vi "Custom Aggregation (1D DBL Array).vi"(0 "data in":dbl[](array[numeric]), 1 "reset? (F)":bool, 5 "aggregation settings":T1={"interval"=1, "interval unit"=enum."Runs", "synchronization of intervals"=enum."Not synchronized", "algorithm"=enum."Average"}, 9 "system info in":refnum<class "EP System Info.lvclass">, 11 "error in (no error)":errorcluster, 12 "data timestamp":timestamp) -> (4 "aggregated minimum values":dbl[](array[numeric]), 6 "aggregated averaged/RMS values":dbl[](array[numeric]), 8 "aggregated maximum values":dbl[](array[numeric]), 10 "system info out":refnum<class "EP System Info.lvclass">, 13 "aggregated data valid?":bool, 14 "aggregated data timestamp":timestamp, 15 "error out":errorcluster)   [LabVIEW 2014, in "NI_EP_Power Quality.lvlib"]
doc: "Calculates the aggregated minimum, maximum, and averaged or RMS value of an input signal for a specified aggregation interval, according to Class S in IEC 61000-4-30:2008. There is no overlap between aggregation intervals. This VI automatically restarts accumulation at the beginning of the next time interval after the previous interval expires. You must manually select the polymorphic instance you want to use.\n\nThis VI supports measuring single-line and multiple-line systems except the DBL instance. Use the DBL instance to measure one channel on one line at one time."
uses:
  <vilib>/addons/Electrical Power/PQ/NI_EP_Power Quality.lvlib
  <vilib>/addons/Electrical Power/PQ/Common/Controls/ep_Aggregation Settings.ctl
  <vilib>/addons/Electrical Power/PQ/Common/Classes/System Info/EP System Info.lvclass
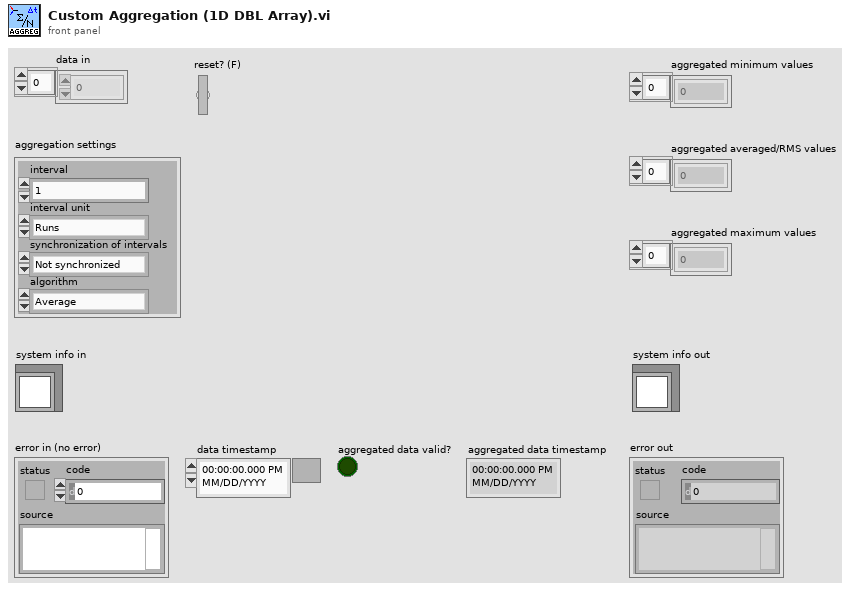
[diagram p1: front panel]
types:
  T1 = typedef "NI_EP_Power Quality.lvlib/ep_Aggregation Settings.ctl" = cluster{"interval":u32, "interval unit":enum16{"Runs", "Seconds", "Minutes", "Hours", "Days", "Weeks"}, "synchronization of intervals":enum16{"Not synchronized", "Interval rounded"}, "algorithm":enum16{"Average", "RMS"}}
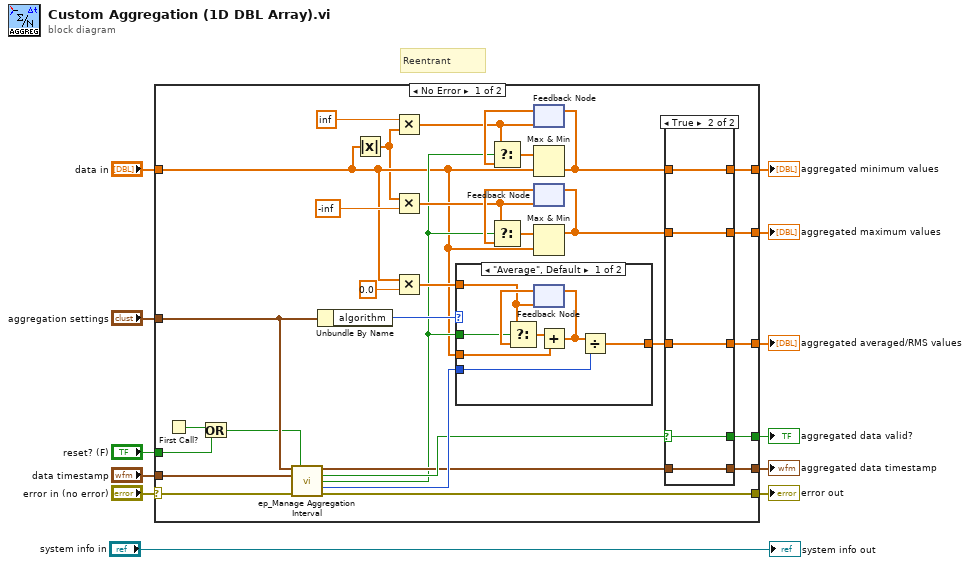
[diagram p0: block diagram]
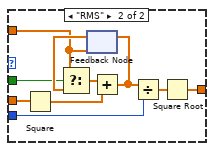
[diagram p3: hidden frame]
diagram:
  # "Reentrant"
  n1 = case shown="No Error" "error in (no error)" {
    selector: "error in (no error)" -> [w27 w69]
    tunnel: "data in" -> [w14 _]
    tunnel: "aggregation settings" -> [w19 _]
    tunnel: "data timestamp" -> [w39 _]
    tunnel: [w37 w69] -> w11
    tunnel: [w26 _] -> w9
    tunnel: [w35 _] -> w6
    tunnel: [w31 _] -> w8
    tunnel: [w30 _] -> w7
    tunnel: [w28 _] -> w10
    tunnel: "reset? (F)" -> [w16 _]
    frame No Error {
      n2 = First Call?() -> (First Call?: T/F=w17:bool)
      n3 = Or(x=w17, y=w16) -> (x .or. y?=w15:bool)
      n4 = call <vilib>:"ep_Manage Aggregation Interval.vi"("aggregation settings"=w19, "restart (F)"=w15, "data time stamp"=w39, "error in (no error)"=w27) -> ("aggregated data time stamp"=w29:timestamp, "aggregated data valid?"=w36:bool, "restart aggregation?"=w18:bool, "runs"=w38:u32, "error out"=w37:errorcluster)  [unwired: 7 in]
      n5 = Unbundle By Name(w19) -> ("algorithm"=w40:enum16{"Average", "RMS"})
      n6 = Absolute Value(x=w14) -> (abs(x)=w13:dbl[])
      n7 = Multiply(x=inf, y=w13) -> (x*y=w24:dbl[])
      n8 = Multiply(x=w13, y=-inf) -> (x*y=w22:dbl[])
      n9 = Multiply(x=w14, y=0.0) -> (x*y=w20:dbl[])
      n10 = case shown="\"Average\", Default" w40 {
        tunnel: w14 -> [w53 w63]
        tunnel: w18 -> [w54 w64]
        tunnel: w38 -> [w58 w68]
        tunnel: [w57 w60] -> w34
        tunnel: w20 -> [w51 w59]
        frame "Average", Default {
          n11 = feedback #1(w51) -> (w56:dbl[])
          n12 = Select(t=w51, s=w54, f=w56) -> (s? t:f=w55:dbl[])
          n13 = Add(x=w55, y=w53) -> (x+y=w52:dbl[])
          n14 = feedback-in #1(w52) -> ()
          n15 = Divide(x=w52, y=w58) -> (x/y=w57:dbl[])
        }
        frame "RMS" {
          n16 = Square(x=w63) -> (x^2=w61:dbl[])
          n17 = feedback #2(w59) -> (w66:dbl[])
          n18 = Select(t=w59, s=w64, f=w66) -> (s? t:f=w65:dbl[])
          n19 = Add(x=w65, y=w61) -> (x+y=w62:dbl[])
          n20 = feedback-in #2(w62) -> ()
          n21 = Divide(x=w62, y=w68) -> (x/y=w67:dbl[])
          n22 = Square Root(x=w67) -> (sqrt(x)=w60:dbl[])
        }
      }
      n23 = feedback #3(w24) -> (w44:dbl[])
      n24 = Select(t=w24, s=w18, f=w44) -> (s? t:f=w43:dbl[])
      n25 = Max & Min(x=w43, y=w14) -> (min(x,y)=w32:dbl[])  [unwired: 1 out]
      n26 = feedback-in #3(w32) -> ()
      n27 = feedback #4(w22) -> (w41:dbl[])
      n28 = Select(t=w22, s=w18, f=w41) -> (s? t:f=w42:dbl[])
      n29 = Max & Min(x=w42, y=w14) -> (max(x,y)=w33:dbl[])  [unwired: 1 out]
      n30 = feedback-in #4(w33) -> ()
      n31 = case shown="True" w36 {
        selector: w36 -> [w45 w46]
        tunnel: [_ w50] -> w35
        tunnel: w34 -> [_ w50]
        tunnel: w33 -> [_ w48]
        tunnel: w32 -> [_ w49]
        tunnel: [_ w49] -> w31
        tunnel: [_ w48] -> w30
        tunnel: w29 -> [_ w47]
        tunnel: [_ w47] -> w28
        tunnel: [w45 w46] -> w26
        frame False {
        }
        frame True {
        }
      }
    }
    frame Error {
    }
  }
  "error out" <- w11
  "aggregated minimum values" <- w8
  "aggregated averaged/RMS values" <- w6
  "aggregated maximum values" <- w7
  "aggregated data valid?" <- w9
  "aggregated data timestamp" <- w10
  "system info out" <- "system info in"
